vi "Render.vi"(7 "Renderer":refnum<class "Renderer.lvclass">, 8 "error in (no error)":errorcluster, 10 "Camera":refnum<class "Camera.lvclass">, 11 "Laser in":refnum<class "Laser.lvclass">) -> (0 "error out":errorcluster)   [LabVIEW 2021, in "Laser.lvclass"]
uses:
  Laser.lvclass
  Camera/Camera.lvclass
  Renderer/Renderer.lvclass
  Laser.lvclass/Laser.ctl
  LabSDL2/Source/Libraries/LibSDL2 Wrapper/LibSDL2.lvlib
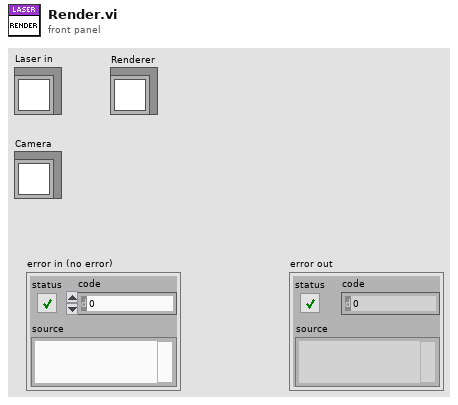
[diagram p1: front panel]
types:
  T1 = typedef "LibSDL2.lvlib/Rectangle.ctl" = cluster{"x":i32, "y":i32, "Width":i32, "Height":i32}
  T2 = typedef "SDL2 Utility.lvlib/Point (I32).ctl" = cluster{"x":i32, "y":i32}
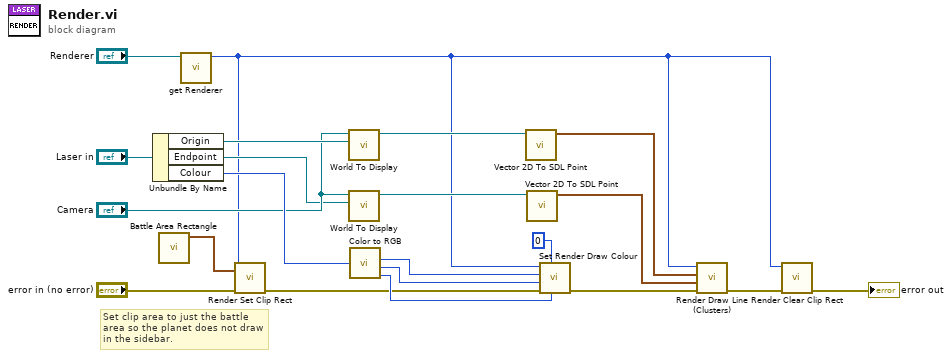
[diagram p0: block diagram]
diagram:
  # "Set clip area to just the battle area so the planet does not draw in the sidebar."
  n1 = Unbundle By Name("Laser in") -> ("Origin"=w13:refnum<class "Vector 2D.lvclass">, "Endpoint"=w11:refnum<class "Vector 2D.lvclass">, "Colour"=w14:u32)
  n2 = call "Battle Area Rectangle.vi"() -> ("Viewport"=w6:T1)  [unwired: 11 in]
  n3 = call-dynamic "get Renderer.vi"("Renderer in"="Renderer") -> ("Renderer"=w1:u32)  [unwired: 10 in]
  n4 = call "Render Set Clip Rect.vi"("error in"="error in (no error)", "Rectangle"=w6, "Renderer Pointer"=w1) -> ("error out"=w4:errorcluster)  [unwired: 7 in, 1 out]
  n5 = call "World To Display.vi"("World Position"=w13, "Camera in"="Camera") -> ("Display Position"=w10:refnum<class "Vector 2D.lvclass">)  [unwired: 9 in]
  n6 = call "World To Display.vi"("World Position"=w11, "Camera in"="Camera") -> ("Display Position"=w8:refnum<class "Vector 2D.lvclass">)  [unwired: 9 in]
  n7 = call <vilib>:"Color to RGB.vi"("Color"=w14) -> ("R"=w18:u8, "G"=w17:u8, "B"=w16:u8)  [unwired: 1 out]
  n8 = call "Vector 2D To SDL Point.vi"("Vector 2D in"=w10) -> ("Point"=w9:T2)  [unwired: 10 in]
  n9 = call "Vector 2D To SDL Point.vi"("Vector 2D in"=w8) -> ("Point"=w7:T2)  [unwired: 10 in]
  n10 = call "Set Render Draw Colour.vi"("B"=w16, "A"=u8 0, "error in (no error)"=w4, "G"=w17, "R"=w18, "Renderer Pointer"=w1) -> ("error out"=w15:errorcluster)  [unwired: 4 in, 1 out]
  n11 = call "Render Draw Line (Clusters).vi"("error in"=w15, "End"=w7, "Start"=w9, "Renderer Pointer"=w1) -> ("error out"=w3:errorcluster)  [unwired: 6 in, 1 out]
  n12 = call "Render Clear Clip Rect.vi"("error in"=w3, "Renderer Pointer"=w1) -> ("error out"=→"error out":errorcluster)  [unwired: 8 in, 1 out]
